vi "test_Multiple Local Comparison Channel Command-Response Messages using Trigger and Padding.vi"(8 "error in (no error)":errorcluster, 11 "TestCase in":refnum<class "Common System Tests.lvclass">) -> (0 "error out":errorcluster, 3 "TestCase out":refnum<class "Common System Tests.lvclass">)   [LabVIEW 2018, in "Common System Tests.lvclass"]
uses:
  Common System Tests.lvclass
  <vilib>/addons/_JKI Toolkits/VI Tester/TestCase.llb/TestCase.lvclass
  <vilib>/NI VeriStand/Execution/Workspace/NI_VS Workspace ExecutionAPI.lvlib
  <vilib>/NI VeriStand/Execution/Workspace/NI VeriStand - Get Multiple Channel Values.vi
  <vilib>/NI VeriStand/Execution/Workspace/NI VeriStand - Set Multiple Channel Values.vi
  C:/Program Files (x86)/National Instruments/LabVIEW 2019/vi.lib/addons/_JKI Toolkits/VI Tester/TestCase.llb/TestCase.lvclass
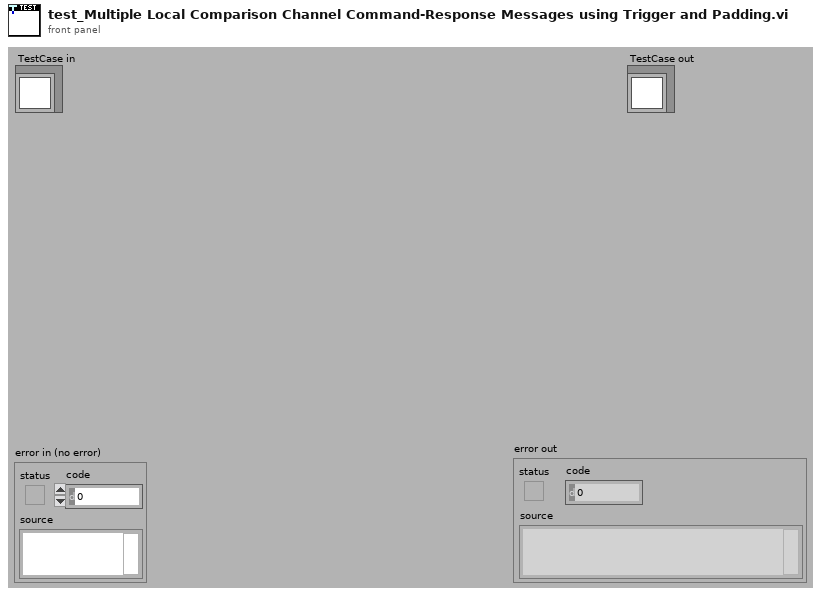
[diagram p1: front panel]
types:
  T1 = typedef "NI_VS Workspace ExecutionAPI.lvlib/WorkspaceAPI.ctl" = refnum<k24>
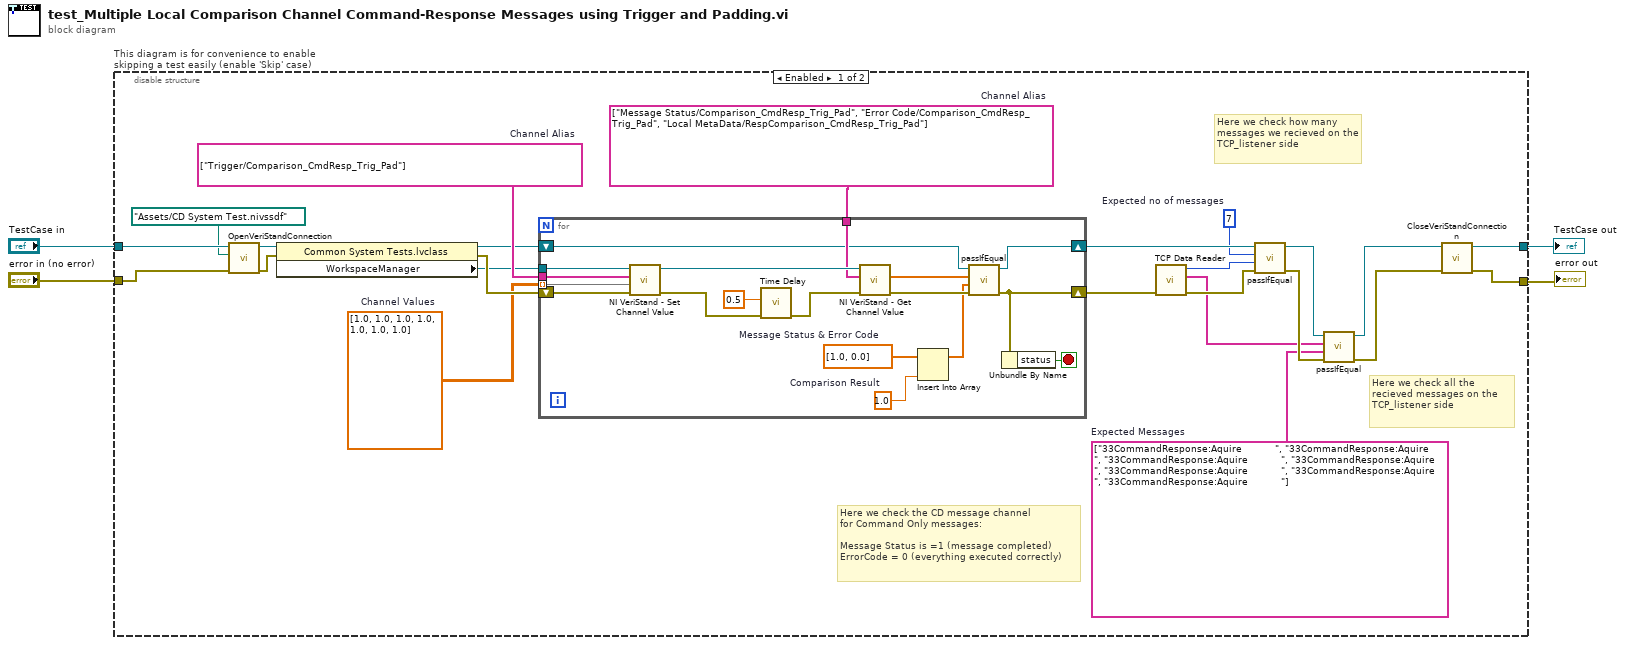
[diagram p0: block diagram]
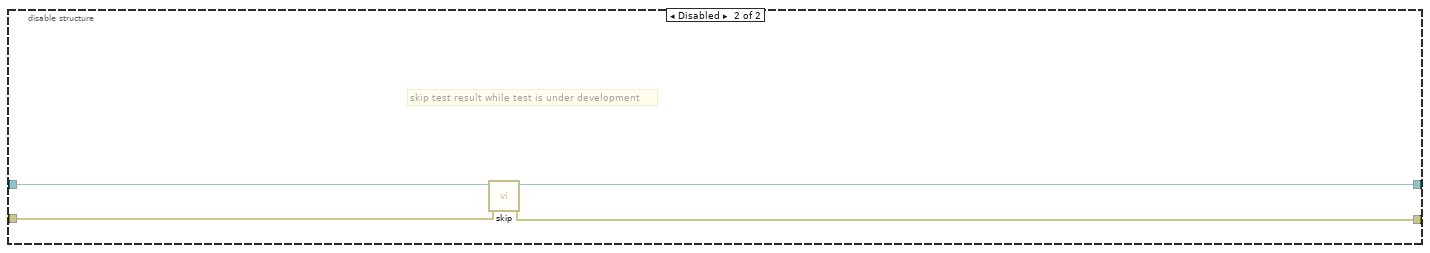
[diagram p2: hidden frame]
diagram:
  n1 = disable-structure "This diagram is for convenience to enable skipping a test easily (enable 'Skip' case)" shown="Enabled" {
    disable-tunnel: "TestCase in" -> [w26 w50]
    disable-tunnel: [w27 w48] -> w1
    disable-tunnel: [w28 w49] -> w3
    disable-tunnel: "error in (no error)" -> [w24 w47]
    frame Enabled {
      w5 = string[] ["33CommandResponse:Aquire           ", "33CommandResponse:Aquire           ", "33CommandResponse:Aquire           ", "33CommandResponse:Aquire           ", "33CommandResponse:Aquire           ", "33CommandResponse:Aquire           ", "33CommandResponse:Aquire           "]  # Expected Messages
      w8 = 7  # Expected no of messages
      w17 = string[] ["Message Status/Comparison_CmdResp_Trig_Pad", "Error Code/Comparison_CmdResp_Trig_Pad", "Local MetaData/RespComparison_CmdResp_Trig_Pad"]  # Channel Alias
      w19 = dbl[][] [[1.0], [1.0], [1.0], [1.0], [1.0], [1.0], [1.0]]  # Channel Values
      w20 = string[] ["Trigger/Comparison_CmdResp_Trig_Pad"]  # Channel Alias
      # "Here we check how many messages we recieved on the TCP_listener side"
      # "Here we check all the recieved messages on the TCP_listener side"
      # "Here we check the CD message channel\nfor Command Only messages:\n\nMessage Status is =1 (message completed)\nErrorCode = 0 (everything executed correctly)"
      n2 = call-dynamic "OpenVeriStandConnection.vi"("error in (no error)"=w24, "System Definition File"=path "Assets/CD System Test.nivssdf", "VeriStand Test Case in"=w26) -> ("error out"=w23:errorcluster, "VeriStand Test Case out"=w25:refnum<class "Common System Tests.lvclass">)  [unwired: 6 in, 1 out]
      n3 = property class="Common System Tests.lvclass"(reference=w25, error in=w23) -> (reference out=w18:refnum<class "Common System Tests.lvclass">, error out=w21:errorcluster, "WorkspaceManager"=w16:T1)
      n4 = for {
        tunnel: w16 -> [w46]
        tunnel: w20 -> [w44]
        tunnel: w19 -> [w32] mode=indexing
        shift-right: [w34] -> w7
        shift-left: w21 -> [w45]
        tunnel: w17 -> [w42]
        shift-right: [w37] -> w15
        shift-left: w18 -> [w38]
        stop <- w33 stop-if-true
        w29 = 1.0  # Comparison Result
        w31 = dbl[] [1.0, 0.0]  # Message Status & Error Code
        n5 = call-poly <vilib>:"NI VeriStand - Set Channel Value.vi"("error in (no error)"=w45, "Values"=w32, "Channels"=w44, "WorkspaceManager in"=w46) -> ("error out"=w40:errorcluster, "WorkspaceManager out"=w43:T1)  [unwired: 6 in]
        n6 = call "Time Delay"("error in (no error)"=w40, "Delay Time (s)"=0.5) -> ("error out"=w39:errorcluster)  [unwired: 9 in]
        n7 = call-poly <vilib>:"NI VeriStand - Get Channel Value.vi"("error in (no error)"=w39, "Channels"=w42, "WorkspaceManager in"=w43) -> ("error out"=w36:errorcluster, "Values"=w35:dbl[])  [unwired: 6 in, 1 out]
        n8 = Insert Into Array(array=w31, new element=w29) -> (w30:dbl[])  [unwired: 1 in]
        n9 = call-dynamic "passIfEqual.vi"("error in (no error)"=w36, "y"=w30, "x"=w35, "TestCase in"=w38) -> ("error out"=w34:errorcluster, "TestCase out"=w37:refnum<class "Common System Tests.lvclass">)  [unwired: 6 in]
        n10 = Unbundle By Name(w34) -> ("status"=w33:bool)
      }
      n11 = call "TCP Data Reader.vi"("error in (no error)"=w7) -> ("error out"=w13:errorcluster, "Recieved Messages"=w6:string[], "No of messages"=w9:i32)  [unwired: 8 in]
      n12 = call-dynamic "passIfEqual.vi"("error in (no error)"=w13, "y"=w9, "x"=w8, "TestCase in"=w15) -> ("error out"=w11:errorcluster, "TestCase out"=w14:refnum<class "Common System Tests.lvclass">)  [unwired: 6 in]
      n13 = call-dynamic "passIfEqual.vi"("error in (no error)"=w11, "y"=w5, "x"=w6, "TestCase in"=w14) -> ("error out"=w10:errorcluster, "TestCase out"=w12:refnum<class "Common System Tests.lvclass">)  [unwired: 6 in]
      n14 = call-dynamic "CloseVeriStandConnection.vi"("error in (no error)"=w10, "VeriStand Test Case in"=w12) -> ("error out"=w28:errorcluster, "VeriStand Test Case out"=w27:refnum<class "Common System Tests.lvclass">)  [unwired: 8 in]
    }
    frame Disabled {
      # "skip test result while test is under development"
      n15 = call <vilib>:"skip.vi"("error in (no error)"=w47, "TestCase in"=w50) -> ("error out"=w49:errorcluster, "TestCase out"=w48:refnum<class "Common System Tests.lvclass">)  [unwired: 8 in]
    }
  }
  "error out" <- w3
  "TestCase out" <- w1
